vi "Bring to front.vi"(8 "错误输入（无错误）":errorcluster) -> (0 "错误输出":errorcluster)   [LabVIEW 2012, in "Application.lvlib"]
uses:
  Application.lvlib
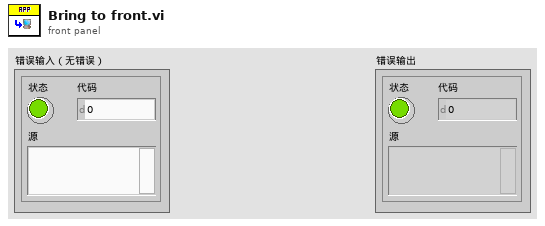
[diagram p1: front panel]
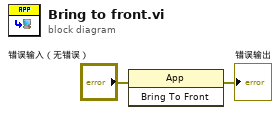
[diagram p0: block diagram]
diagram:
  n1 = invoke class="App" method="Bring To Front"(error in="错误输入（无错误）") -> (error out=→"错误输出":errorcluster)  [unwired: 2 in, 2 out]
